vi "Raised Cosine Filter.vi"() -> ()   [LabVIEW 2023]
doc: "Demonstrates how to use the DFD Raised Cosine Design VI to design a raised cosine finite impulse response (FIR) filter.\n\nComplete the following steps to use this VI.\n1) Run the VI.\n2) Change the values of the <B>Samples per Symbol</B> and <B>Filter Length</B> inputs and run this VI again.\n3) Observe the Coefficients and Magnitude Response graphs. Notice that the coefficients equal zero at every <B>Samples per Symbol</B> location, except for the middle coefficient.\n4) Change the <B>Roll Off</B> value and run this VI again to view the transition band changes."
uses:
  <vilib>/addons/Digital Filter Design/_Objects.llb/DFD Multirate Filtering Mode.ctl
  <vilib>/addons/Digital Filter Design/NI_DigFilterLicensed.lvlib
panel:
  out "Error Message":string
  out "Coefficients":dbl[](graph)
  out "Magnitude Response":cluster{"f0":dbl, "df":dbl, "values":dbl[]}[](graph)
  in  "Window":u16(ring)=1 items=["None"=0, "Hanning"=1, "Hamming"=2, "Blackman-Harris"=3, "Exact Blackman"=4, "Blackman"=5, "Flat Top"=6, "4 Term B-Harris"=7, "7 Term B-Harris"=8, "Low Sidelobe"=9, "Triangular"=30]
  in  "Roll Off":dbl=0.25
  in  "Samples per Symbol":i32=4
  in  "Filter Length [Symbols]":i32=11
  # "Select Help>>Show Context Help and move the cursor over the VI icon for more information."
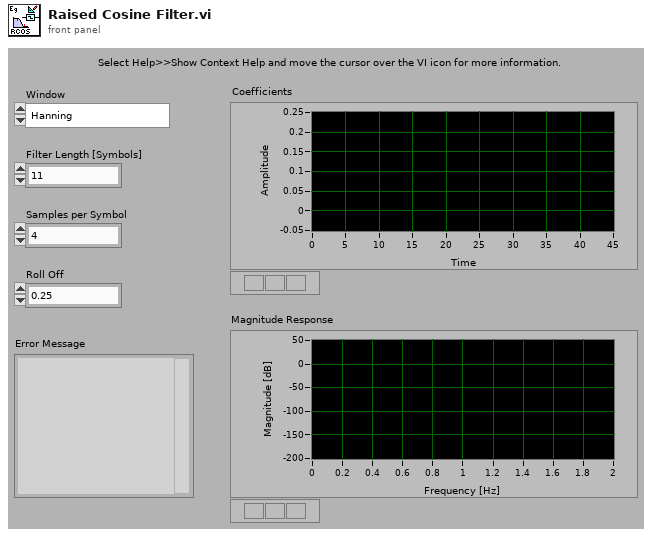
[diagram p1: front panel]
types:
  T1 = typedef "NI_DigFilterLicensed.lvlib/DFD Multirate Filtering Mode.ctl" = u16
  T2 = typedef "NI_DigFilterLicensed.lvlib/DFD Multirate Filter Obj.ctl" = cluster{"mMRate_Structure":enum16{"CIC", "FIR", "IIR", "Lattice"}, "mMRate_Mode":T3, "mMRate_Factor":i32, "mMRate_FIRParams":cluster{"mMRate_FIR_H":dbl[], "mMRate_FIR_IsNyquist?":bool, "mMRate_FIR_IsSymmetric?":bool}, "mMRate_CICParams":cluster{"mMRate_CIC_#Stage":i32, "mMRate_CIC_Lag":i32, "mMRate_CIC_Type":enum16{"Lowpass", "Highpass"}}, "mMRate_Order":i32, "mMRate_Version":string, "mMRate_Comments":string, "mMRate_RationalFactor":cluster{"mMRate_L":i32, "mMRate_M":i32}, "mMRate_Fs":dbl, "mMRate_Quantized?":bool, "mMRate_QFilterGain":dbl, "mMRate_CoefWl":i16, "mMRate_Scaling":cluster{"mMRate_ScaleByPowerOf2?":bool, "mMRate_ScaleType":T4}, "mMRate_InputWl":i16, "mMRate_OutputWl":i16, "mMRate_OutputMode":T5, "mMRate_MultMode":T6, "mMRate_BitPruning":bool, "mMRate_GainWl":i16, "mMRate_OutputFwl":i16, "mMRate_SumIwl":i16, "mMRate_InputIwl ":i16, "mMRate_SumWl":i16, "mMRate_CoefIwl":i16}
  T3 = typedef "NI_DigFilterLicensed.lvlib/DFD Multirate Mode.ctl" = i16
  T4 = typedef "NI_DigFilterLicensed.lvlib/DFD Coef Norm Type.ctl" = enum16{"No Norm", "Time Domain 1-Norm", "Time Domain 2-Norm", "Time Domain Inf-Norm"}
  T5 = typedef "NI_DigFilterLicensed.lvlib/DFD Round-off Mode.ctl" = enum16{"Nearest", "Truncation"}
  T6 = typedef "NI_DigFilterLicensed.lvlib/DFD FXP MRate Multiply Mode.ctl" = enum16{"Truncated", "Full"}
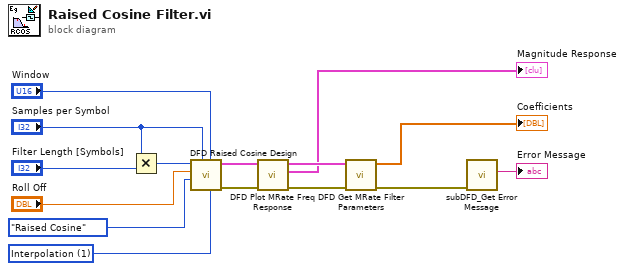
[diagram p0: block diagram]
diagram:
  w3 = T1 1 items=["No Rate Change", "Interpolation", "Decimation"] ("filtering mode")
  n1 = Multiply(x="Samples per Symbol", y="Filter Length [Symbols]") -> (x*y=w12:i32)
  n2 = call <vilib>:"DFD Raised Cosine Design.vi"("filtering mode"=w3, "window"="Window", "factor"="Samples per Symbol", "type"=enum16{"Raised Cosine", "Root Raised Cosine"}."Raised Cosine" ("filter type"), "roll off"="Roll Off", "order"=w12) -> ("error out"=w4:errorcluster, "multirate filter out"=w5:T2)  [unwired: 2 in, 2 out]
  n3 = call <vilib>:"DFD Plot MRate Freq Response.vi"("error in (no error)"=w4, "multirate filter in"=w5) -> ("error out"=w8:errorcluster, "magnitude response"=→"Magnitude Response":cluster{"f0":dbl, "df":dbl, "values":dbl[]}[], "multirate filter out"=w7:T2)  [unwired: 5 in, 2 out]
  n4 = call <vilib>:"DFD Get MRate Filter Parameters.vi"("error in (no error)"=w8, "multirate filter in"=w7) -> ("error out"=w1:errorcluster, "h(n)"=→"Coefficients":dbl[])  [unwired: 1 in, 7 out]
  n5 = call <vilib>:"subDFD_Get Error Message.vi"("error in (no error)"=w1) -> ("Error Message"=→"Error Message":string)  [unwired: 10 out]
